vi "TURCK GUI TestPanel AO.vi"() -> ()   [LabVIEW 2021]
doc: "example for writing values to the TBEN-S2-4AO modul from Turck"
uses:
  KH TURCK ETHERNETIP TDefCluster TBEN-S2-4AO Input Values.ctl
  KH EthernetIP 17.19/KH_EthernetIP_Globals.vi
panel:
  out "TBEN-S2-4AO Input Values":T1
  in  "AO3":u16(slide) scale=0.0..65535.0
  in  "AO2":u16(slide) scale=0.0..65535.0
  in  "AO1":u16(slide) scale=0.0..65535.0
  in  "AO0":u16(slide) scale=0.0..65535.0
  out "error out":errorcluster
  in  "Exit":bool
  # "- Before starting the VI your PC has to be in the same subnet as the modules"
  # "Kirschenhofer Maschinen GmbH\nRömerstraße 35, 89278 Nersingen-Straß\ninfo@kirschenhofer-gmbh.de"
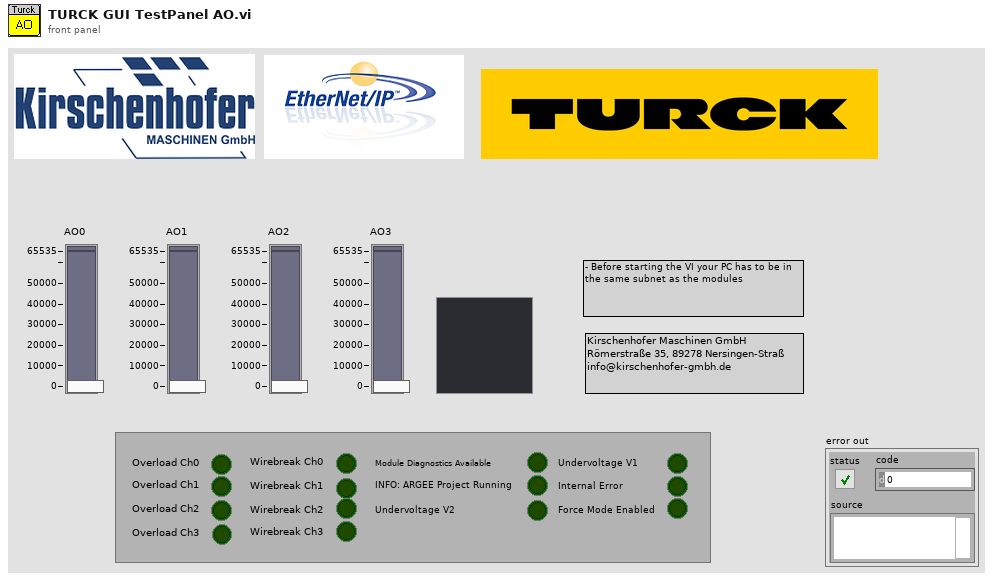
[diagram p1: front panel]
types:
  T1 = typedef "KH TURCK ETHERNETIP TDefCluster TBEN-S2-4AO Input Values.ctl" = cluster{"Overload Ch0":bool, "Overload Ch1":bool, "Overload Ch2":bool, "Overload Ch3":bool, "Wirebreak Ch0":bool, "Wirebreak Ch1":bool, "Wirebreak Ch2":bool, "Wirebreak Ch3":bool, "Module Diagnostics Available":bool, "INFO: ARGEE Project Running":bool, "Undervoltage V2":bool, "Undervoltage V1":bool, "Internal Error":bool, "Force Mode Enabled":bool}
  T2 = cluster{"ItemCount":u16, "AdressItem":cluster{"TypeID":u16, "Length":u16, "Data":cluster{"ConnectionIdentifier":u32, "SequenceNumber":u32}}, "DataItem":cluster{"TypeID":u16, "Length":u16, "Data":u8[], "Sequence Count":u16}}
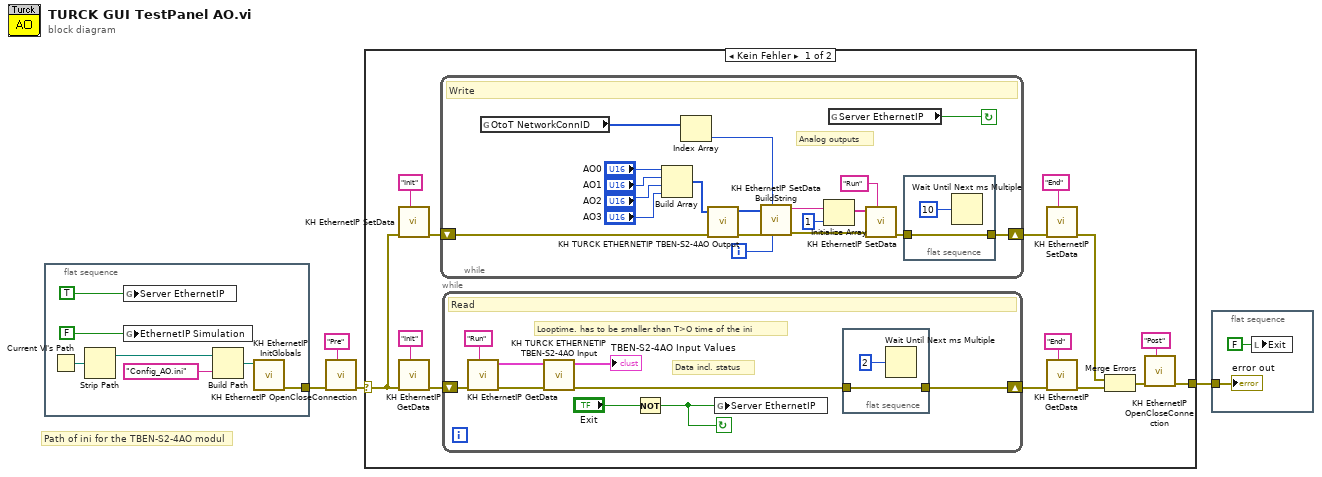
[diagram p0: block diagram]
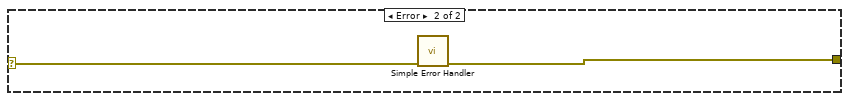
[diagram p2: hidden frame]
diagram:
  # "Path of ini for the TBEN-S2-4AO modul"
  n1 = flat-sequence {
    tunnel: [w11] -> w2
    frame #0 {
      n2 = Current VI's Path() -> (path=w6:path)
      n3 = Strip Path(path=w6) -> (stripped path=w9:path)  [unwired: 1 out]
      n4 = global write "KH_EthernetIP_Globals.vi" "Server EthernetIP"(TRUE ("Server EthernetIP")) -> ()
      n5 = global write "KH_EthernetIP_Globals.vi" "EthernetIP Simulation"(FALSE ("EthernetIP Simulation")) -> ()
      n6 = Build Path(base path=w9, name or relative path="Config_AO.ini") -> (appended path=w7:path)
      n7 = call "KH EthernetIP InitGlobals.vi"("Config File"=w7) -> ("err out"=w11:errorcluster)  [unwired: 10 in]
    }
  }
  n8 = call "KH EthernetIP OpenCloseConnection.vi"("Function"="Pre", "error in"=w2) -> ("error out"=w1:errorcluster)  [unwired: 9 in]
  n9 = case shown="Kein Fehler" w1 {
    selector: w1 -> [w12 w59]
    tunnel: [w13 w58] -> w3
    frame No Error {
      n10 = call "KH EthernetIP SetData.vi"("Function"="Init", "error in"=w12) -> ("error out"=w24:errorcluster)  [unwired: 7 in, 2 out]
      n11 = call "KH EthernetIP GetData.vi"("Function"="Init", "error in"=w12) -> ("error out"=w14:errorcluster)  [unwired: 8 in, 1 out]
      n12 = while {
        shift-right: [w42] -> w23
        shift-left: w24 -> [w33]
        i -> [w36]
        stop <- w41 continue-if-true
        # "Analog outputs"
        # "Write"
        n13 = global read "KH_EthernetIP_Globals.vi" "OtoT NetworkConnID"() -> (w27:u32[])
        n14 = Build Array("AO0", "AO1", "AO2", "AO3") -> (w29:u16[])
        n15 = Index Array(array=w27) -> (element=w26:u32)  [unwired: 1 in]
        n16 = call "KH TURCK ETHERNETIP TBEN-S2-4AO Output.vi"("error in"=w33, "TBEN-S2-4AO Output Values"=w29) -> ("error out"=w34:errorcluster, "Output Data"=w39:u8[])  [unwired: 8 in]
        n17 = call "KH EthernetIP SetData BuildString.vi"("LoopIndex"=w36, "OtoT NetworkConnID"=w26, "error in"=w34, "Output Data"=w39) -> ("error out"=w35:errorcluster, "DataString"=w40:string)  [unwired: 6 in]
        n18 = Initialize Array(w40, 1 ("dimension size")) -> (w37:string[])
        n19 = global read "KH_EthernetIP_Globals.vi" "Server EthernetIP"() -> (w41:bool)
        n20 = call "KH EthernetIP SetData.vi"("Function"="Run", "error in"=w35, "Data Strings"=w37) -> ("error out"=w43:errorcluster)  [unwired: 6 in, 2 out]
        n21 = flat-sequence {
          tunnel: w43 -> [w45]
          tunnel: [w45] -> w42
          frame #0 {
            n22 = Wait Until Next ms Multiple(millisecond multiple=u32 10) -> ()  [unwired: 1 out]
          }
        }
      }
      n23 = while {
        shift-right: [w53] -> w16
        shift-left: w14 -> [w55]
        stop <- w51 continue-if-true
        # "Looptime. has to be smaller than T>O time of the ini"
        # "Data incl. status"
        # "Read"
        n24 = call "KH EthernetIP GetData.vi"("Function"="Run", "error in"=w55) -> ("error out"=w49:errorcluster, "Response Data"=w50:T2)  [unwired: 8 in]
        n25 = call "KH TURCK ETHERNETIP TBEN-S2-4AO Input.vi"("error in"=w49, "Response Data"=w50) -> ("error out"=w48:errorcluster, "TBEN-S2-4AO Input Values"=→"TBEN-S2-4AO Input Values":T1)  [unwired: 8 in]
        n26 = Not(x="Exit") -> (.not. x?=w51:bool)
        n27 = global write "KH_EthernetIP_Globals.vi" "Server EthernetIP"(w51) -> ()
        n28 = flat-sequence {
          tunnel: w48 -> [w56]
          tunnel: [w56] -> w53
          frame #0 {
            n29 = Wait Until Next ms Multiple(millisecond multiple=u32 2) -> ()  [unwired: 1 out]
          }
        }
      }
      n30 = call "KH EthernetIP SetData.vi"("Function"="End", "error in"=w23) -> ("error out"=w19:errorcluster)  [unwired: 7 in, 2 out]
      n31 = call "KH EthernetIP GetData.vi"("Function"="End", "error in"=w16) -> ("error out"=w21:errorcluster)  [unwired: 8 in, 1 out]
      n32 = Merge Errors(w19, w21) -> (w20:errorcluster)
      n33 = call "KH EthernetIP OpenCloseConnection.vi"("Function"="Post", "error in"=w20) -> ("error out"=w13:errorcluster)  [unwired: 9 in]
    }
    frame Error {
      n34 = call <vilib>:"Simple Error Handler.vi"("error in (no error)"=w59) -> ("error out"=w58:errorcluster)  [unwired: 4 in, 4 out]
    }
  }
  n35 = flat-sequence {
    tunnel: w3 -> [w60]
    frame #0 {
      n36 = local write "Exit"(FALSE ("Exit")) -> ()
      "error out" <- w60
    }
  }
